vi "DAC Stop.vi"(8 "error in":errorcluster, 11 "DAC FTCU in":refnum<class "DAC FTCU.lvclass">) -> (0 "error out":errorcluster, 3 "DAC FTCU out":refnum<class "DAC FTCU.lvclass">)   [LabVIEW 2019, in "DAC.lvlib" / "DAC FTCU.lvclass"]
uses:
  DAC FTCU.lvclass
  C:/Users/wg/Documents/LV_Projects/test-stand/App/DAC/DAC.lvclass
  DAC.lvclass/DAC.ctl
  DAC FTCU.lvclass/DAC FTCU.ctl
  <vilib>/NI/Modbus Library/API/Master/Modbus Master.lvclass
  DAC.lvclass
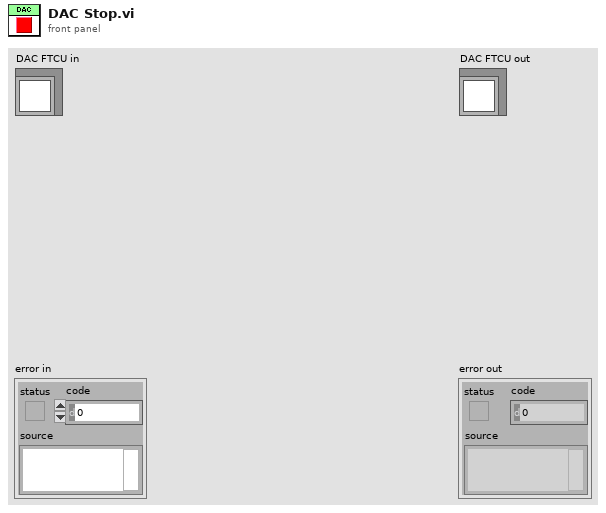
[diagram p1: front panel]
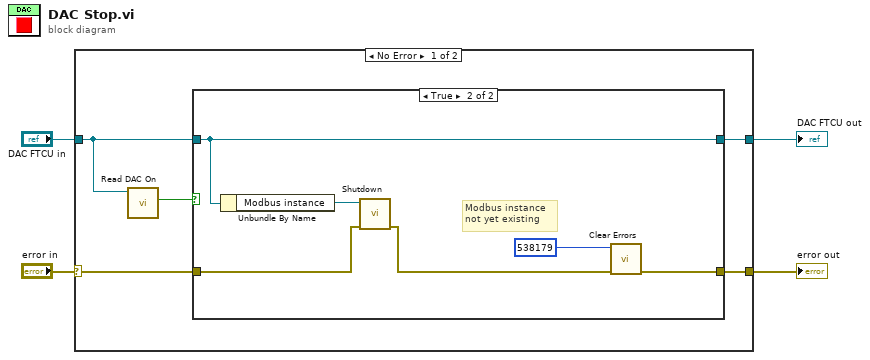
[diagram p0: block diagram]
diagram:
  n1 = case shown="No Error" "error in" {
    selector: "error in" -> [w6 w19]
    tunnel: [w5 w19] -> w1
    tunnel: [w7 w18] -> w3
    tunnel: "DAC FTCU in" -> [w9 w18]
    frame No Error {
      n2 = call "Read DAC On.vi"("DAC in"=w9) -> ("DAC On"=w8:bool)  [unwired: 8 in, 2 out]
      n3 = case shown="True" w8 {
        tunnel: w9 -> [w11 w17]
        tunnel: [w11 w17] -> w7
        tunnel: w6 -> [w10 w15]
        tunnel: [w10 w13] -> w5
        frame False {
        }
        frame True {
          # "Modbus instance\nnot yet existing"
          n4 = Unbundle By Name(w17) -> ("Modbus instance"=w16:refnum<class "Modbus Master.lvclass">)
          n5 = call-dynamic "Shutdown.vi"("error in"=w15, "Modbus master in"=w16) -> ("error out"=w14:errorcluster)  [unwired: 9 in]
          n6 = call <vilib>:"Clear Errors.vi"("error in (no error)"=w14, "specific error code to clear (0: all)"=538179) -> ("error out"=w13:errorcluster)  [unwired: 4 in, 1 out]
        }
      }
    }
    frame Error {
    }
  }
  "error out" <- w1
  "DAC FTCU out" <- w3
